vi "insert values.vi"(4 "数据库类型":T2, 5 "是否创建唯一键":bool, 6 "Password":string, 7 "data":variant[](array[variant]), 8 "错误输入（无错误）":errorcluster, 9 "columns外部输入":T1, 10 "database":string="database1", 11 "Tabe Name":string) -> (0 "错误输出":errorcluster)   [LabVIEW 2016]
uses:
  Access/Access Lib.lvlib
  SQLite/SQLite Lib.lvlib
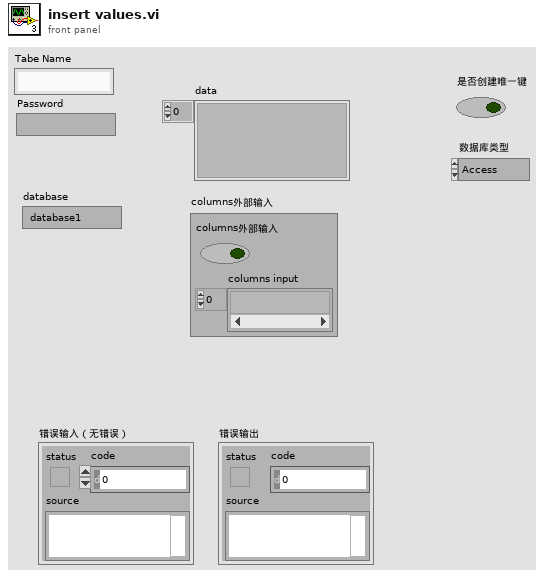
[diagram p1: front panel]
types:
  T1 = cluster{"columns外部输入":bool, "columns input":string[]}
  T2 = typedef "数据库类型.ctl" = enum16{"Access", "SQLite"}
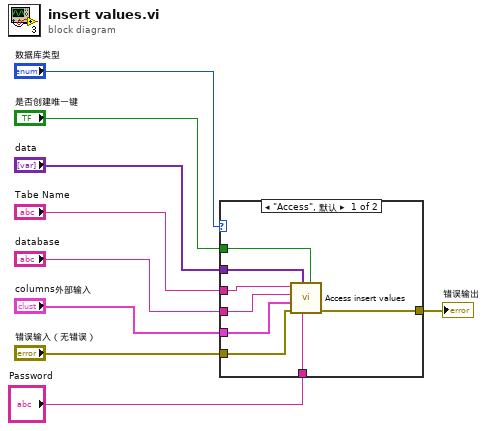
[diagram p0: block diagram]
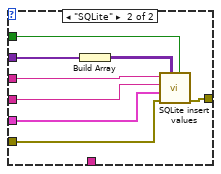
[diagram p2: hidden frame]
diagram:
  n1 = case shown="\"Access\", 默认" "数据库类型" {
    tunnel: "Tabe Name" -> [w13 w25]
    tunnel: "是否创建唯一键" -> [w16 w24]
    tunnel: "错误输入（无错误）" -> [w15 w23]
    tunnel: [w14 w22] -> w6
    tunnel: "data" -> [w17 w21]
    tunnel: "database" -> [w12 w19]
    tunnel: "columns外部输入" -> [w11 w18]
    tunnel: "Password" -> [w10 _]
    frame "Access", Default {
      n2 = call "Access insert values.vi"("是否创建唯一键"=w16, "Password"=w10, "data"=w17, "error in (no error)"=w15, "columns外部输入"=w11, "database"=w12, "table"=w13) -> ("error out"=w14:errorcluster)  [unwired: 4 in]
    }
    frame "SQLite" {
      n3 = Build Array(w21) -> (w20:variant[][])
      n4 = call "SQLite insert values.vi"("是否创建唯一键"=w24, "数组"=w20, "错误输入（无错误）"=w23, "columns外部输入"=w18, "database"=w19, "Tabe Name"=w25) -> ("错误输出"=w22:errorcluster)  [unwired: 5 in]
    }
  }
  "错误输出" <- w6
